vi "JJMCclase11p2.vi"() -> ()   [LabVIEW 2013]
uses:
  <vilib>/express/express arith-compare/Formula/XNode/ExpressFormulaBlockNode.xnode
panel:
  out "OBS":string
  in  "Finalizar":bool
  in  "GenerarImPar":bool
  out "Numero ImPar":dbl
  in  "GenerarPar":bool
  out "Numero Par":dbl
  # "Usando eventos generar un numero par al presionar un GenerarPar y generar\nun numero impar al presionar un numero ImPar"
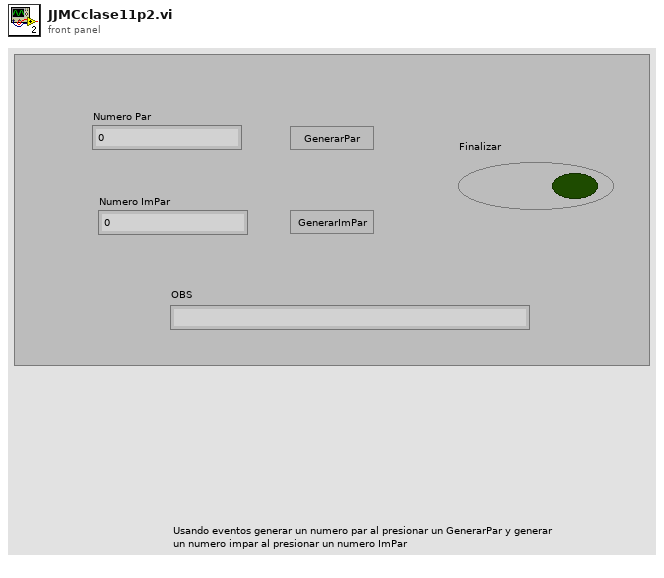
[diagram p1: front panel]
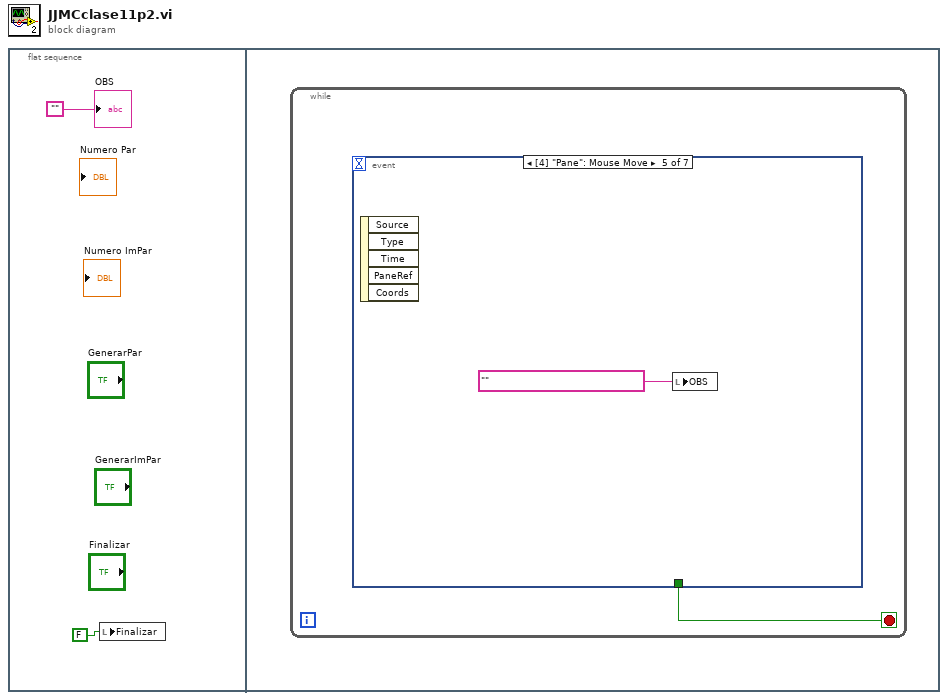
[diagram p0: block diagram]
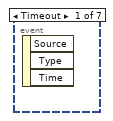
[diagram p2: hidden frame]
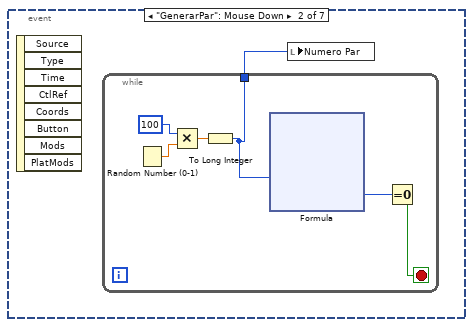
[diagram p3: hidden frame]
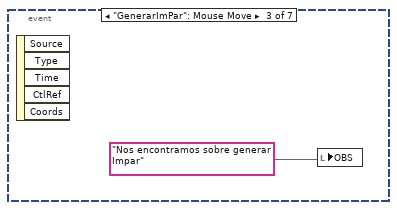
[diagram p4: hidden frame]
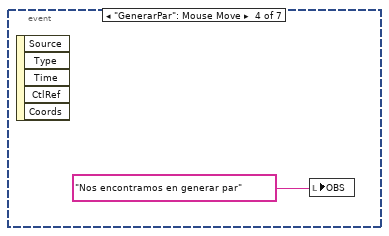
[diagram p5: hidden frame]
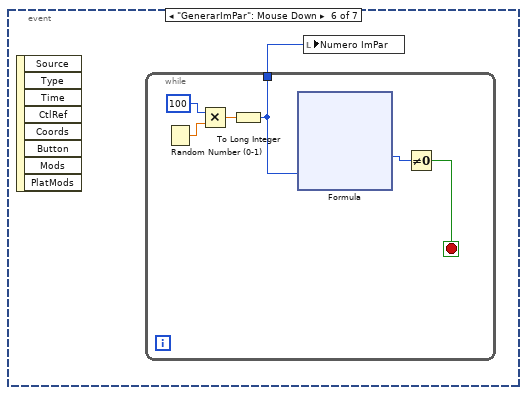
[diagram p6: hidden frame]
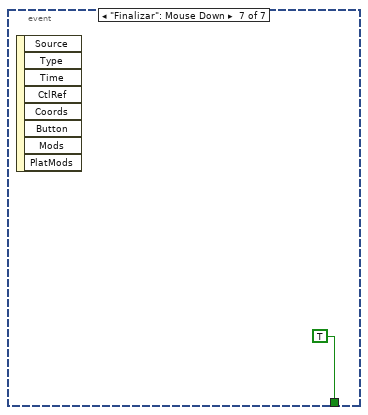
[diagram p7: hidden frame]
diagram:
  n1 = flat-sequence {
    frame #0 {
      n2 = local write "Finalizar"(FALSE) -> ()
      "OBS" <- ""
    }
    frame #1 {
      n3 = while {
        stop <- w3 stop-if-true
        n4 = event shown="[4] \"Pane\": Mouse Move" {
          selector: _ -> [_ _ _ _ _ _ _]
          dyn-events: _ -> [_ _ _ _ _ _ _]
          timeout: _ -> [_ _ _ _ _ _ _]
          tunnel: [_ _ _ _ _ _ TRUE] -> w3
          event Timeout {
            n5 = event-data() -> ()  [unwired: 1 in, 3 out]
          }
          event "GenerarPar": Mouse Down {
            n6 = event-data() -> ()  [unwired: 1 in, 8 out]
            n7 = while {
              tunnel: [w5] -> w4
              stop <- w6 stop-if-true
              n8 = Random Number (0-1)() -> (number: 0 to 1=w9:dbl)
              n9 = Multiply(x=100, y=w9) -> (x*y=w8:dbl)
              n10 = To Long Integer(number=w8) -> (32bit integer=w5:i32)
              n11 = xnode "Formula"("X1"=w5) -> ("Result"=w7:i32)  [unwired: 1 in, 1 out]
              n12 = Equal To 0?(x=w7) -> (x = 0?=w6:bool)
            }
            n13 = local write "Numero Par"(w4) -> ()
          }
          event "GenerarImPar": Mouse Move {
            n14 = event-data() -> ()  [unwired: 1 in, 5 out]
            n15 = local write "OBS"("Nos encontramos sobre generar Impar") -> ()
          }
          event "GenerarPar": Mouse Move {
            n16 = event-data() -> ()  [unwired: 1 in, 5 out]
            n17 = local write "OBS"("Nos encontramos en generar par") -> ()
          }
          event Mouse Move {
            n18 = event-data() -> ()  [unwired: 1 in, 5 out]
            n19 = local write "OBS"("") -> ()
          }
          event "GenerarImPar": Mouse Down {
            n20 = event-data() -> ()  [unwired: 1 in, 8 out]
            n21 = while {
              tunnel: [w25] -> w22
              stop <- w23 stop-if-true
              n22 = Random Number (0-1)() -> (number: 0 to 1=w27:dbl)
              n23 = Multiply(x=100, y=w27) -> (x*y=w26:dbl)
              n24 = To Long Integer(number=w26) -> (32bit integer=w25:i32)
              n25 = xnode "Formula"("X1"=w25) -> ("Result"=w24:i32)  [unwired: 1 in, 1 out]
              n26 = Not Equal To 0?(x=w24) -> (x != 0?=w23:bool)
            }
            n27 = local write "Numero ImPar"(w22) -> ()
          }
          event "Finalizar": Mouse Down {
            n28 = event-data() -> ()  [unwired: 1 in, 8 out]
          }
        }
      }
    }
  }
